vi "UE9 Quadrature.vi"(8 "error in":errorcluster) -> (0 "error out":errorcluster)   [LabVIEW 2021]
panel:
  in  "Case Constant\n(See Context Help)":bool=TRUE
  in  "DeviceType":u16(ring)=1 items=["LJ_dtU3", "LJ_dtUE9"]
  in  "Stop":bool
  in  "Reset Count":bool
  out "Quadrature Count":i32
  in  "FirstFound":bool=TRUE
  in  "Address":string="1"
  in  "ConnectionType":u16(ring) items=["LJ_ctUSB", "LJ_ctETHERNET"]
  out "Error Message":string
  # "Demonstrates 1 quadrature input, which uses two timer channels for phases A and B (FIO0 and FIO1 in this case).\nIf you don't have a quadrature signal source handy, you can connect wires to GND, and tap these wires on FIO0\nand FIO1 to simulate quadrature."
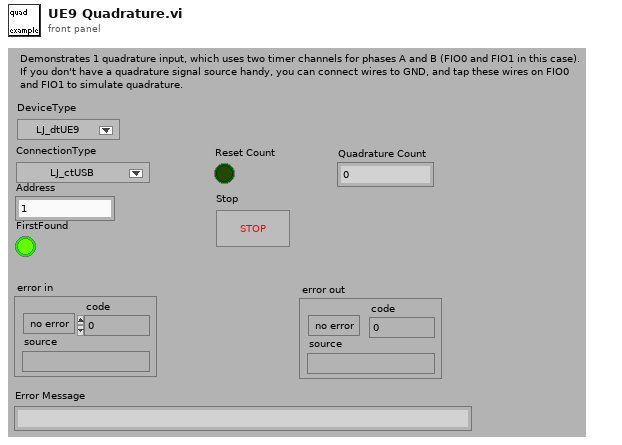
[diagram p1: front panel]
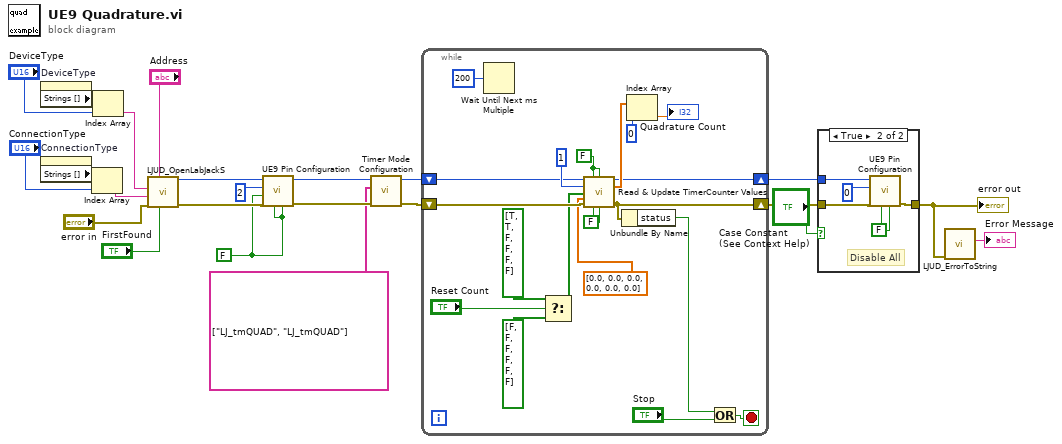
[diagram p0: block diagram]
diagram:
  w2 = FALSE ("Enable Counter0")
  n1 = property on="DeviceType" class="Ring (strict)"() -> ("Strings []"=w10:string[])  [unwired: 2 in, 2 out]
  n2 = property on="ConnectionType" class="Ring (strict)"() -> ("Strings []"=w12:string[])  [unwired: 2 in, 2 out]
  n3 = Index Array(array=w12, index="ConnectionType") -> (element=w11:string)
  n4 = Index Array(array=w10, index="DeviceType") -> (element=w8:string)
  n5 = call "LJUD_OpenLabJackS.vi"("FirstFound"="FirstFound", "Address"="Address", "error in"="error in", "ConnectionType"=w11, "DeviceType"=w8) -> ("error out"=w5:errorcluster, "Handle"=w4:i32)  [unwired: 4 in, 1 out]
  n6 = call "UE9 Pin Configuration.vi"("Enable Counter1"=w2, "Enable Counter0"=w2, "error in"=w5, "Enable DACs"=w2, "Number of Timers Enabled"=2 ("# Timers Enabled"), "Handle In"=w4) -> ("error out"=w6:errorcluster, "Handle Out"=w3:i32)  [unwired: 4 in]
  n7 = call "Timer Mode Configuration.vi"("error in"=w6, "TimerModes"=string[] ["LJ_tmQUAD", "LJ_tmQUAD"], "Handle In"=w3) -> ("error out"=w17:errorcluster, "Handle Out"=w16:i32)  [unwired: 7 in]
  n8 = while {
    shift-right: [w35] -> w14
    shift-left: w16 -> [w37]
    shift-right: [w30] -> w15
    shift-left: w17 -> [w36]
    stop <- w29 stop-if-true
    w24 = FALSE ("Reset Counter0")
    w42 = FALSE ("Reset Counter0")
    n9 = Wait Until Next ms Multiple(millisecond multiple=u32 200) -> ()  [unwired: 1 out]
    n10 = Select(t=bool[] [TRUE, TRUE, FALSE, FALSE, FALSE, FALSE] ("UpdateReset Timers"), s="Reset Count", f=bool[] [FALSE, FALSE, FALSE, FALSE, FALSE, FALSE] ("UpdateReset Timers")) -> (s? t:f=w31:bool[])
    n11 = call "Read & Update TimerCounter Values.vi"("Handle In"=w37, "Reset Counter0"=w42, "Reset Counter1"=w42, "# Timers to Read"=1, "UpdateReset Timers"=w31, "TimerValues"=dbl[] [0.0, 0.0, 0.0, 0.0, 0.0, 0.0], "error in"=w36, "Read Counter0"=w24, "Read Counter1"=w24) -> ("Handle Out"=w35:i32, "Timer Value Reads"=w38:dbl[], "error out"=w30:errorcluster)  [unwired: 3 in, 1 out]
    n12 = Unbundle By Name(w30) -> ("status"=w28:bool)
    n13 = Index Array(array=w38, index=0 ("Index")) -> (element=→"Quadrature Count":dbl)
    n14 = Or(x=w28, y="Stop") -> (x .or. y?=w29:bool)
  }
  n15 = case shown="True" "Case Constant\n(See Context Help)" {
    tunnel: w15 -> [w43 w48]
    tunnel: w14 -> [_ w47]
    tunnel: [w43 w46] -> w19
    frame False {
    }
    frame True {
      w44 = FALSE ("Enable Counter0")
      # "Disable All"
      n16 = call "UE9 Pin Configuration.vi"("Enable Counter1"=w44, "Enable Counter0"=w44, "error in"=w48, "Number of Timers Enabled"=0 ("# Timers Enabled"), "Handle In"=w47) -> ("error out"=w46:errorcluster)  [unwired: 5 in, 1 out]
    }
  }
  "error out" <- w19
  n17 = call "LJUD_ErrorToString.vi"("error in"=w19) -> ("String"=→"Error Message":string)  [unwired: 10 in]
